vi "lf-condition - 副本.vi"(11 "面板属性":T3(array[cluster]) {"panle"."ID" min=1}) -> ()   [LabVIEW 2019]
panel:
  in  "添加面板":bool
  in  "字符串":string caption="面板地址"
  in  "单选按钮 2":T1(radio)
  in  "树形":string(tree)
  in  "簇 6":T2
  in  "簇 5":T2
  in  "簇 4":T2
  in  "簇 3":T2
  in  "簇 2":T2
  in  "簇 1":T2
  in  "确定按钮 2":bool
  in  "确定按钮":bool
  # "面板ID"
  # "(地址)"
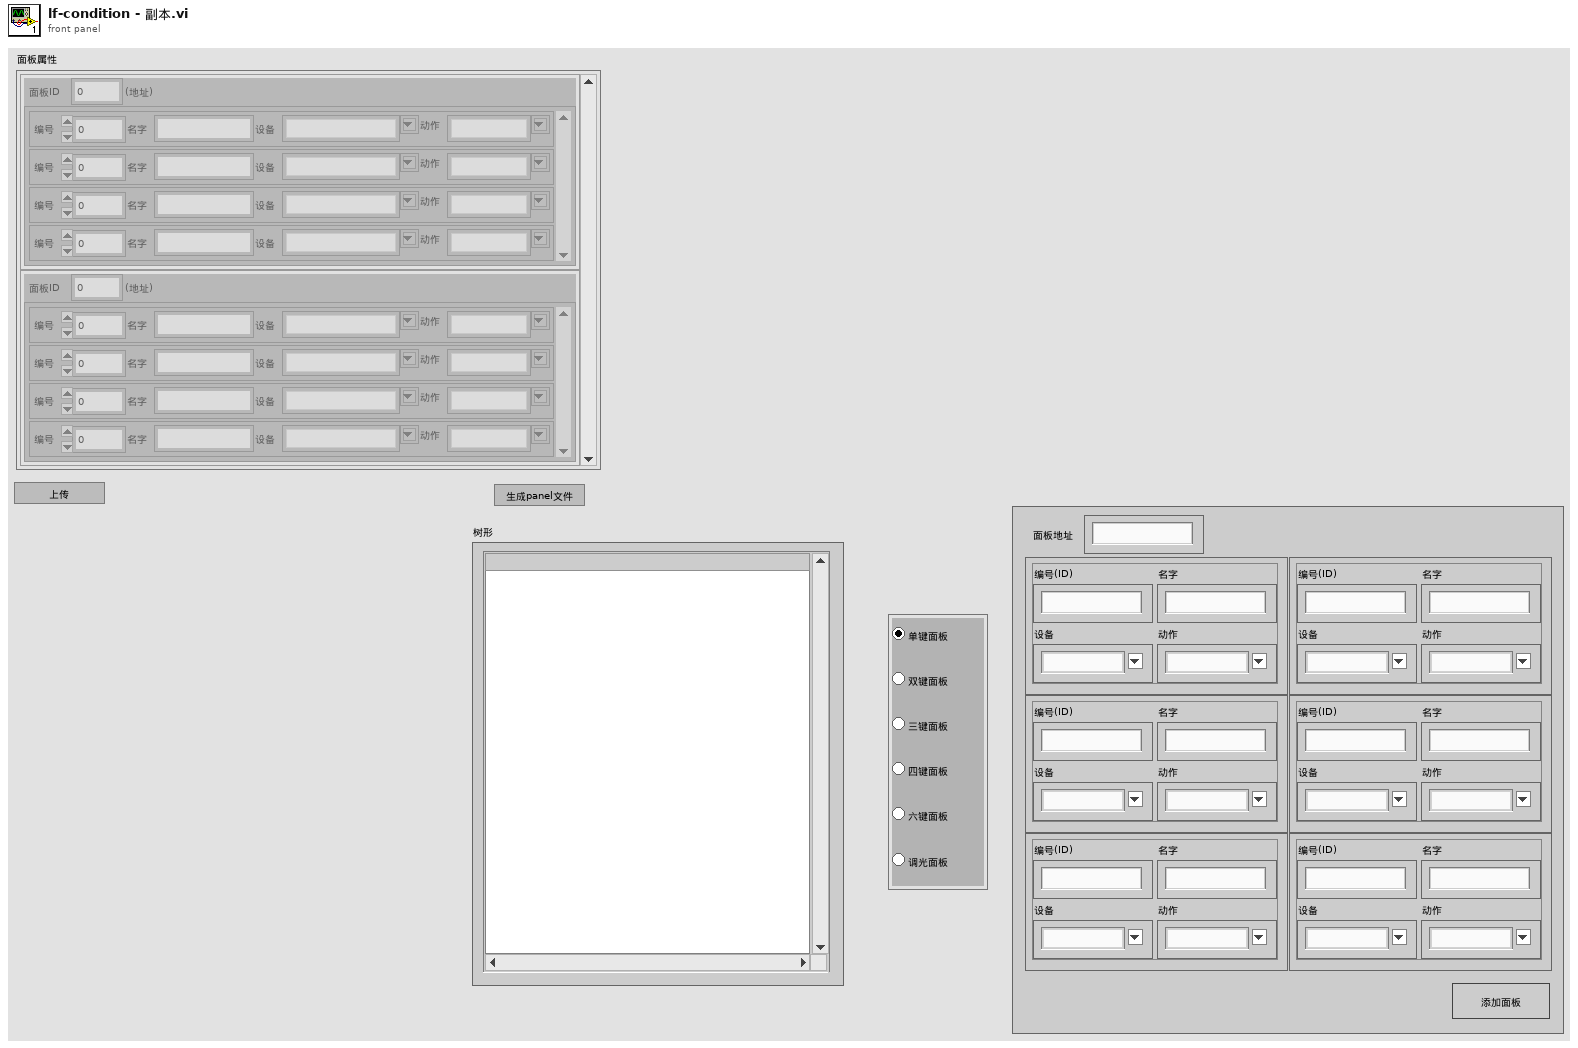
[diagram p1: front panel]
types:
  T1 = enum32{"单键面板", "双键面板", "三键面板", "四键面板", "六键面板", "调光面板"}
  T2 = cluster{"ID":string, "Attribute":string, "Action":string, "name":string}
  T3 = cluster{"id":dbl, "panle":cluster{"ID":u8, "Name":string, "Attribute":string, "Action":string}[]}[]
  T4 = cluster{"ID":u8, "Name":string, "Attribute":string, "Action":string}[]
  T5 = cluster{"id":dbl, "panle":cluster{"ID":u8, "Name":string, "Attribute":string, "Action":string}[]}
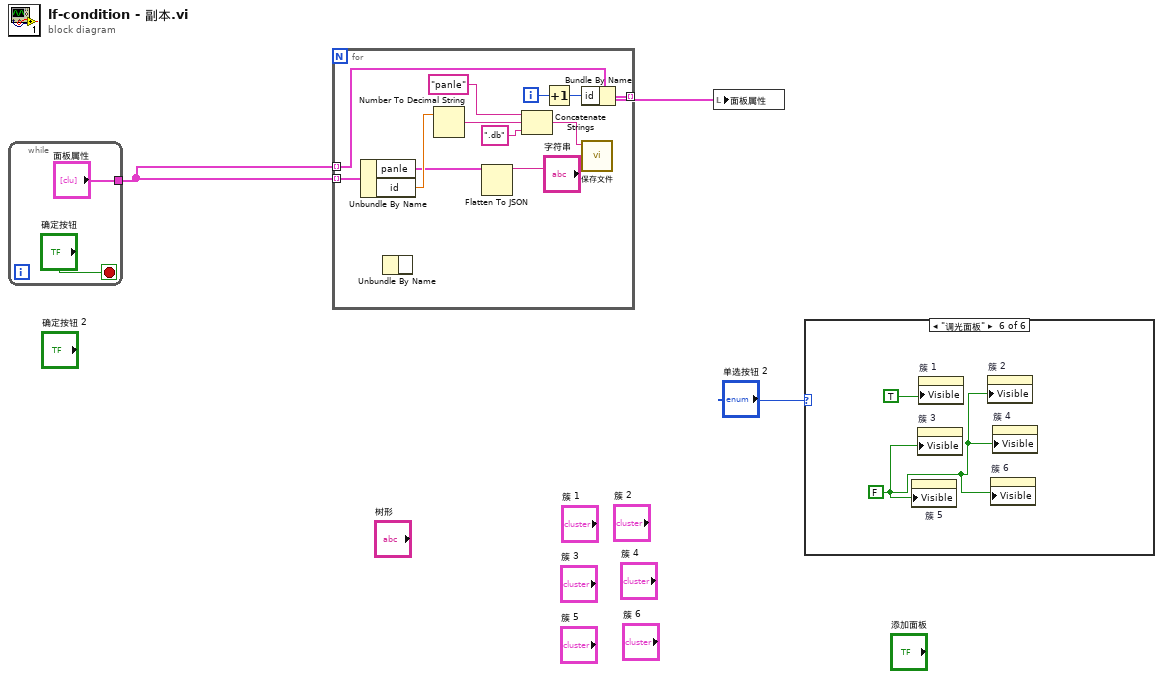
[diagram p0: block diagram]
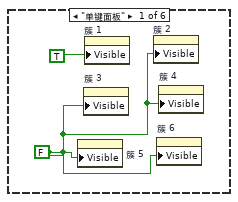
[diagram p2: hidden frame]
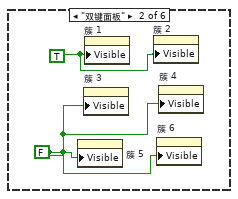
[diagram p3: hidden frame]
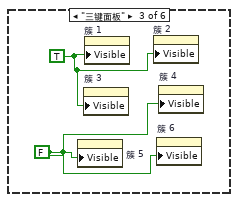
[diagram p4: hidden frame]
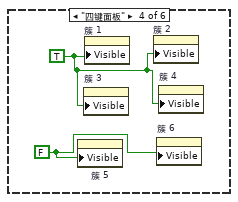
[diagram p5: hidden frame]
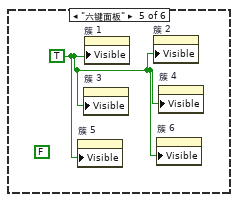
[diagram p6: hidden frame]
diagram:
  n1 = while {
    tunnel: ["面板属性"] -> w3
    stop <- "确定按钮" stop-if-true
  }
  n2 = for {
    tunnel: w3 -> [w17] mode=indexing
    tunnel: [w16] -> w2 mode=indexing
    tunnel: w3 -> [w13] mode=indexing
    i -> [w14]
    n3 = Unbundle By Name(w13) -> ("panle"=w6:T4, "id"=w12:dbl)
    n4 = Unbundle By Name() -> ()  [unwired: 1 in, 1 out]
    n5 = Number To Decimal String(number=w12) -> (decimal integer string=w11:string)  [unwired: 1 in]
    n6 = Flatten To JSON(anything=w6) -> (JSON string=w8:string)  [unwired: 2 in, 1 out]
    n7 = Concatenate Strings("panle", w11, ".db") -> (w7:string)
    n8 = Increment(x=w14) -> (x+1=w15:i32)
    n9 = Bundle By Name(cluster=w17, "id"=w15) -> (w16:T5)
    n10 = call "保存文件.vi"("input"=w8, "文件名"=w7) -> ()  [unwired: 9 in, 1 out]
  }
  n11 = local write "面板属性"(w2) -> ()
  n12 = case shown="\"调光面板\"" "单选按钮 2" {
    frame "单键面板" {
      w18 = FALSE
      n13 = property on="簇 5" class="Clust (严格)"("Visible"=w18) -> ()  [unwired: 2 in, 2 out]
      n14 = property on="簇 3" class="Clust (严格)"("Visible"=w18) -> ()  [unwired: 2 in, 2 out]
      n15 = property on="簇 1" class="Clust (严格)"("Visible"=TRUE) -> ()  [unwired: 2 in, 2 out]
      n16 = property on="簇 2" class="Clust (严格)"("Visible"=w18) -> ()  [unwired: 2 in, 2 out]
      n17 = property on="簇 6" class="Clust (严格)"("Visible"=w18) -> ()  [unwired: 2 in, 2 out]
      n18 = property on="簇 4" class="Clust (严格)"("Visible"=w18) -> ()  [unwired: 2 in, 2 out]
    }
    frame "双键面板" {
      w21 = FALSE
      w20 = TRUE
      n19 = property on="簇 5" class="Clust (严格)"("Visible"=w21) -> ()  [unwired: 2 in, 2 out]
      n20 = property on="簇 3" class="Clust (严格)"("Visible"=w21) -> ()  [unwired: 2 in, 2 out]
      n21 = property on="簇 1" class="Clust (严格)"("Visible"=w20) -> ()  [unwired: 2 in, 2 out]
      n22 = property on="簇 2" class="Clust (严格)"("Visible"=w20) -> ()  [unwired: 2 in, 2 out]
      n23 = property on="簇 6" class="Clust (严格)"("Visible"=w21) -> ()  [unwired: 2 in, 2 out]
      n24 = property on="簇 4" class="Clust (严格)"("Visible"=w21) -> ()  [unwired: 2 in, 2 out]
    }
    frame "三键面板" {
      w23 = FALSE
      w22 = TRUE
      n25 = property on="簇 5" class="Clust (严格)"("Visible"=w23) -> ()  [unwired: 2 in, 2 out]
      n26 = property on="簇 3" class="Clust (严格)"("Visible"=w22) -> ()  [unwired: 2 in, 2 out]
      n27 = property on="簇 1" class="Clust (严格)"("Visible"=w22) -> ()  [unwired: 2 in, 2 out]
      n28 = property on="簇 2" class="Clust (严格)"("Visible"=w22) -> ()  [unwired: 2 in, 2 out]
      n29 = property on="簇 6" class="Clust (严格)"("Visible"=w23) -> ()  [unwired: 2 in, 2 out]
      n30 = property on="簇 4" class="Clust (严格)"("Visible"=w23) -> ()  [unwired: 2 in, 2 out]
    }
    frame "四键面板" {
      w25 = FALSE
      w24 = TRUE
      n31 = property on="簇 5" class="Clust (严格)"("Visible"=w25) -> ()  [unwired: 2 in, 2 out]
      n32 = property on="簇 3" class="Clust (严格)"("Visible"=w24) -> ()  [unwired: 2 in, 2 out]
      n33 = property on="簇 1" class="Clust (严格)"("Visible"=w24) -> ()  [unwired: 2 in, 2 out]
      n34 = property on="簇 2" class="Clust (严格)"("Visible"=w24) -> ()  [unwired: 2 in, 2 out]
      n35 = property on="簇 6" class="Clust (严格)"("Visible"=w25) -> ()  [unwired: 2 in, 2 out]
      n36 = property on="簇 4" class="Clust (严格)"("Visible"=w24) -> ()  [unwired: 2 in, 2 out]
    }
    frame "六键面板" {
      (unwired) FALSE
      w26 = TRUE
      n37 = property on="簇 5" class="Clust (严格)"("Visible"=w26) -> ()  [unwired: 2 in, 2 out]
      n38 = property on="簇 3" class="Clust (严格)"("Visible"=w26) -> ()  [unwired: 2 in, 2 out]
      n39 = property on="簇 1" class="Clust (严格)"("Visible"=w26) -> ()  [unwired: 2 in, 2 out]
      n40 = property on="簇 2" class="Clust (严格)"("Visible"=w26) -> ()  [unwired: 2 in, 2 out]
      n41 = property on="簇 6" class="Clust (严格)"("Visible"=w26) -> ()  [unwired: 2 in, 2 out]
      n42 = property on="簇 4" class="Clust (严格)"("Visible"=w26) -> ()  [unwired: 2 in, 2 out]
    }
    frame "调光面板" {
      w28 = FALSE
      n43 = property on="簇 5" class="Clust (严格)"("Visible"=w28) -> ()  [unwired: 2 in, 2 out]
      n44 = property on="簇 3" class="Clust (严格)"("Visible"=w28) -> ()  [unwired: 2 in, 2 out]
      n45 = property on="簇 1" class="Clust (严格)"("Visible"=TRUE) -> ()  [unwired: 2 in, 2 out]
      n46 = property on="簇 2" class="Clust (严格)"("Visible"=w28) -> ()  [unwired: 2 in, 2 out]
      n47 = property on="簇 6" class="Clust (严格)"("Visible"=w28) -> ()  [unwired: 2 in, 2 out]
      n48 = property on="簇 4" class="Clust (严格)"("Visible"=w28) -> ()  [unwired: 2 in, 2 out]
    }
  }
